vi "TypeSignal.vi"(8 "error in":errorcluster, 10 "SygnalType":T1) -> (0 "error out":errorcluster)   [LabVIEW 2020, in "Settings.lvlib"]
doc: "_____\nCreated using DQMH Event Scripter 6.0.0.122."
uses:
  Settings.lvlib
  AcqType--enum.ctl
  TypeSignal Argument--cluster.ctl
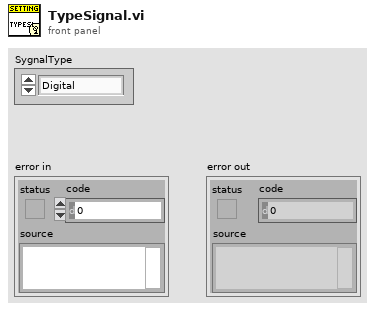
[diagram p1: front panel]
types:
  T1 = typedef "AcqType--enum.ctl" = enum16{"Digital", "Analog"}
  T2 = typedef "Settings.lvlib/TypeSignal Argument--cluster.ctl" = cluster{"SygnalType":T1}
  T3 = typedef "Settings.lvlib/Broadcast Events--cluster.ctl" = cluster{"Module Did Init":refnum<user-event>, "Status Updated":refnum<user-event>, "Error Reported":refnum<user-event>, "Module Did Stop":refnum<user-event>, "Update Module Execution Status":refnum<user-event>, "NameTest":refnum<user-event>, "SecuenceHasBeenSent":refnum<user-event>, "TypeSignal":refnum<user-event>}
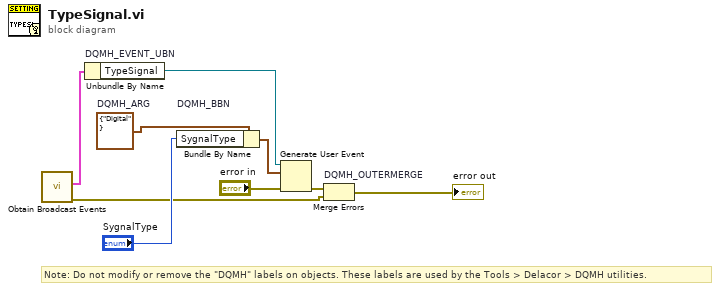
[diagram p0: block diagram]
diagram:
  w4 = T2 {"SygnalType"=enum."Digital"}  # DQMH_ARG
  # "Note: Do not modify or remove the \"DQMH\" labels on objects. These labels are used by the Tools > Delacor > DQMH utilities."
  n1 = call "Obtain Broadcast Events.vi"() -> ("error out"=w2:errorcluster, "Settings Broadcast Events"=w1:T3)  [unwired: 10 in]
  n2 = Unbundle By Name "DQMH_EVENT_UBN"(w1) -> ("TypeSignal"=w6:refnum<user-event>)
  n3 = Bundle By Name "DQMH_BBN"(cluster=w4, "SygnalType"="SygnalType") -> (w7:T2)
  n4 = Generate User Event(user event=w6, event data cluster=w7, error in="error in") -> (error out=w5:errorcluster)  [unwired: 1 in, 1 out]
  n5 = Merge Errors "DQMH_OUTERMERGE"(w5, w2) -> (→"error out":errorcluster)
